vi "translateMotorStatus.vi"(0 "DMXJSAController in":refnum<class "DMXJSAController.lvclass">, 2 "actual value":u32, 5 "error in (no error)":errorcluster) -> (14 "DMXJSAController out":refnum<class "DMXJSAController.lvclass">, 16 "motion_state":T1=enum."CONST", 17 "other_states":T1[](array[typedef]), 19 "error out":errorcluster)   [LabVIEW 2020, in "classes.lvlib" / "DMXJSAController.lvclass"]
doc: "Retrieve the motor status for an attached DMX-J-SA\n\nProduced By:\n\n<B>Kod Integrations, LLC</B>\n4835 Marianne Drive\nMount Airy, MD 21771\nhttp://www.kodintegrations.com\nemail: info@kodintegrations.com\nphone: (240) 687-1288"
uses:
  DMXJSAController.lvclass
  common/controls/motor_status.ctl
  libraries/common.lvlib
panel:
  out "other states":bool[](array[boolean])
  out "motion state":bool[](array[boolean])
  out "actual bits":bool[](array[boolean])
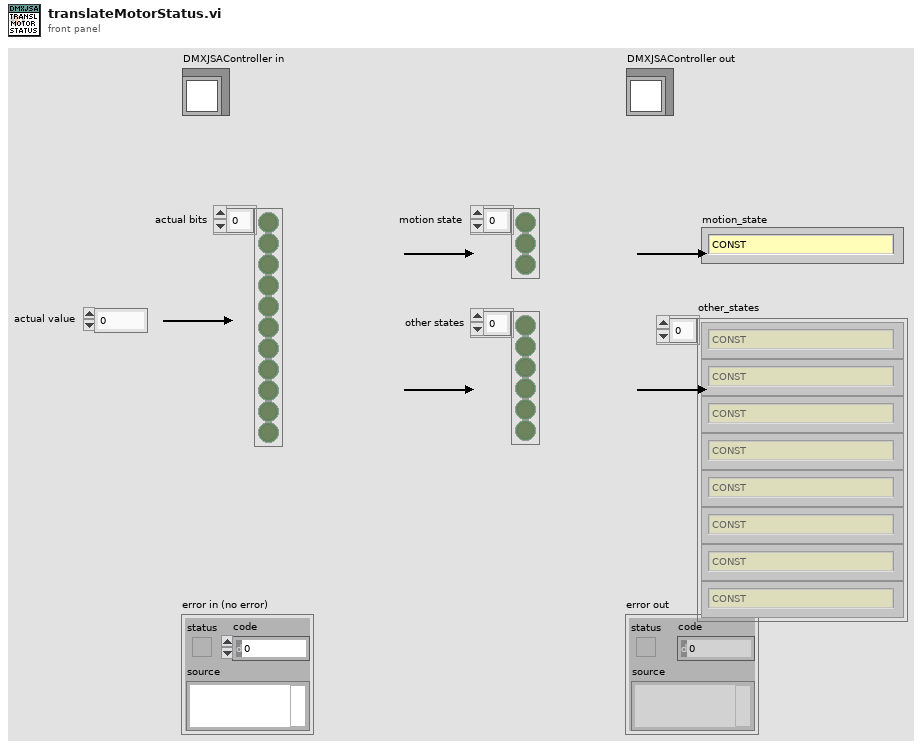
[diagram p1: front panel]
types:
  T1 = typedef "common.lvlib/motor_status.ctl" = enum16{"IDLE", "CONST", "ACCEL", "DECEL", "HOME_SWITCH", "-LIMIT_SWITCH", "+LIMIT_SWITCH", "-LIMIT_ERR", "+LIMIT_ERR", "COMM_TIMEOUT", "ALARM_INPUT", "ALARM_ERROR", "TOC_TIMEOUT_STATUS", "LATCH_INPUT_STATUS", "Z_INDEX_STATUS"}
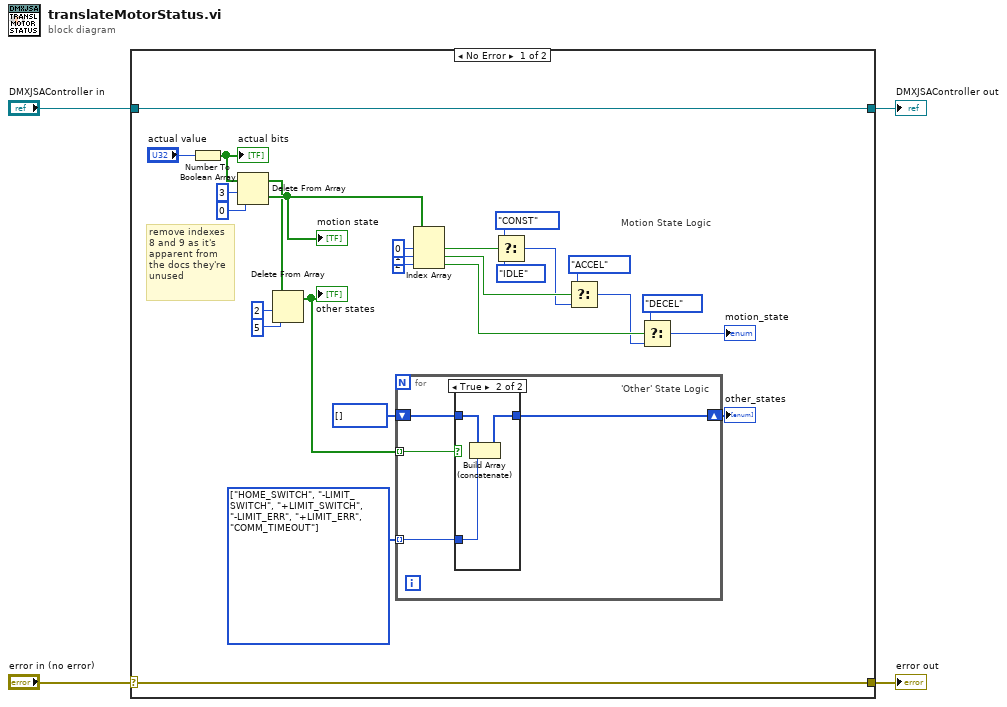
[diagram p0: block diagram]
diagram:
  n1 = case shown="No Error" "error in (no error)" {
    selector: "error in (no error)" -> [w30 w41]
    tunnel: [w30 w41] -> w3
    tunnel: [w31 w40] -> w1
    tunnel: "DMXJSAController in" -> [w31 w40]
    frame No Error {
      w10 = T1[] [enum."HOME_SWITCH", enum."-LIMIT_SWITCH", enum."+LIMIT_SWITCH", enum."-LIMIT_ERR", enum."+LIMIT_ERR", enum."COMM_TIMEOUT"] items=["IDLE", "CONST", "ACCEL", "DECEL", "HOME_SWITCH", "-LIMIT_SWITCH", "+LIMIT_SWITCH", "-LIMIT_ERR", "+LIMIT_ERR", "COMM_TIMEOUT", "ALARM_INPUT", "ALARM_ERROR", "TOC_TIMEOUT_STATUS", "LATCH_INPUT_STATUS", "Z_INDEX_STATUS"]
      w11 = T1[] [] items=["IDLE", "CONST", "ACCEL", "DECEL", "HOME_SWITCH", "-LIMIT_SWITCH", "+LIMIT_SWITCH", "-LIMIT_ERR", "+LIMIT_ERR", "COMM_TIMEOUT", "ALARM_INPUT", "ALARM_ERROR", "TOC_TIMEOUT_STATUS", "LATCH_INPUT_STATUS", "Z_INDEX_STATUS"]
      # "remove indexes\n8 and 9 as it's \napparent from \nthe docs they're\nunused"
      # "Motion State Logic"
      n2 = Number To Boolean Array(number="actual value") -> (Boolean array=w28:bool[])
      "actual bits" <- w28
      n3 = Delete From Array(array=w28, length=3, index=0) -> (deleted portion=w12:bool[], array with subset deleted=w8:bool[])
      "motion state" <- w12
      n4 = Delete From Array(array=w8, length=2, index=5 ("length")) -> (array with subset deleted=w5:bool[])  [unwired: 1 out]
      "other states" <- w5
      n5 = for {
        tunnel: w5 -> [w35] mode=indexing
        shift-right: [w32] -> w9
        shift-left: w11 -> [w34]
        tunnel: w10 -> [w33] mode=indexing
        # "'Other' State Logic"
        n6 = case shown="True" w35 {
          tunnel: w34 -> [w36 w39]
          tunnel: w33 -> [_ w38]
          tunnel: [w36 w37] -> w32
          frame False {
          }
          frame True {
            n7 = Build Array (concatenate)(w39, w38) -> (w37:T1[])
          }
        }
      }
      "other_states" <- w9
      n8 = Index Array(array=w12, index #1=0 ("index"), index #2=1 ("index"), index #3=2 ("index")) -> (element #1=w21:bool, element #2=w19:bool, element #3=w15:bool)
      n9 = Select(t=motor_status."CONST" ("motion_state"), s=w21, f=motor_status."IDLE" ("motion_state")) -> (s? t:f=w18:T1)
      n10 = Select(t=motor_status."ACCEL" ("motion_state"), s=w19, f=w18) -> (s? t:f=w14:T1)
      n11 = Select(t=motor_status."DECEL" ("motion_state"), s=w15, f=w14) -> (s? t:f=→"motion_state":T1)
    }
    frame Error {
    }
  }
  "error out" <- w3
  "DMXJSAController out" <- w1
